vi "main_serce.vi"() -> ()   [LabVIEW 2025]
uses:
  <vilib>/Analysis/8numeric.llb/1D Numeric Integration.vi
  <vilib>/Analysis/NI_AALPro.lvlib
panel:
  out "Data unsaved!":bool
  in  "Save Data":bool
  out "CO value calculated":dbl
  out "Blood temp":dbl
  in  "CO":bool
  out "Waveform Chart":waveform(dbl)(graph)
  out "Bolus Temp":dbl
  in  "Get bolus temp":bool
  in  "Start Measurement":bool
  in  "stop (F)":bool
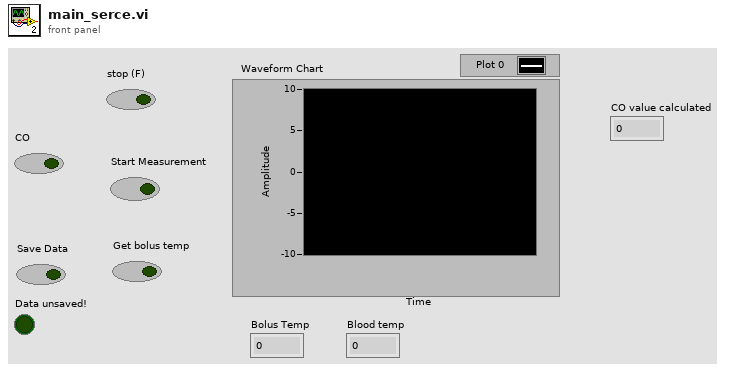
[diagram p1: front panel]
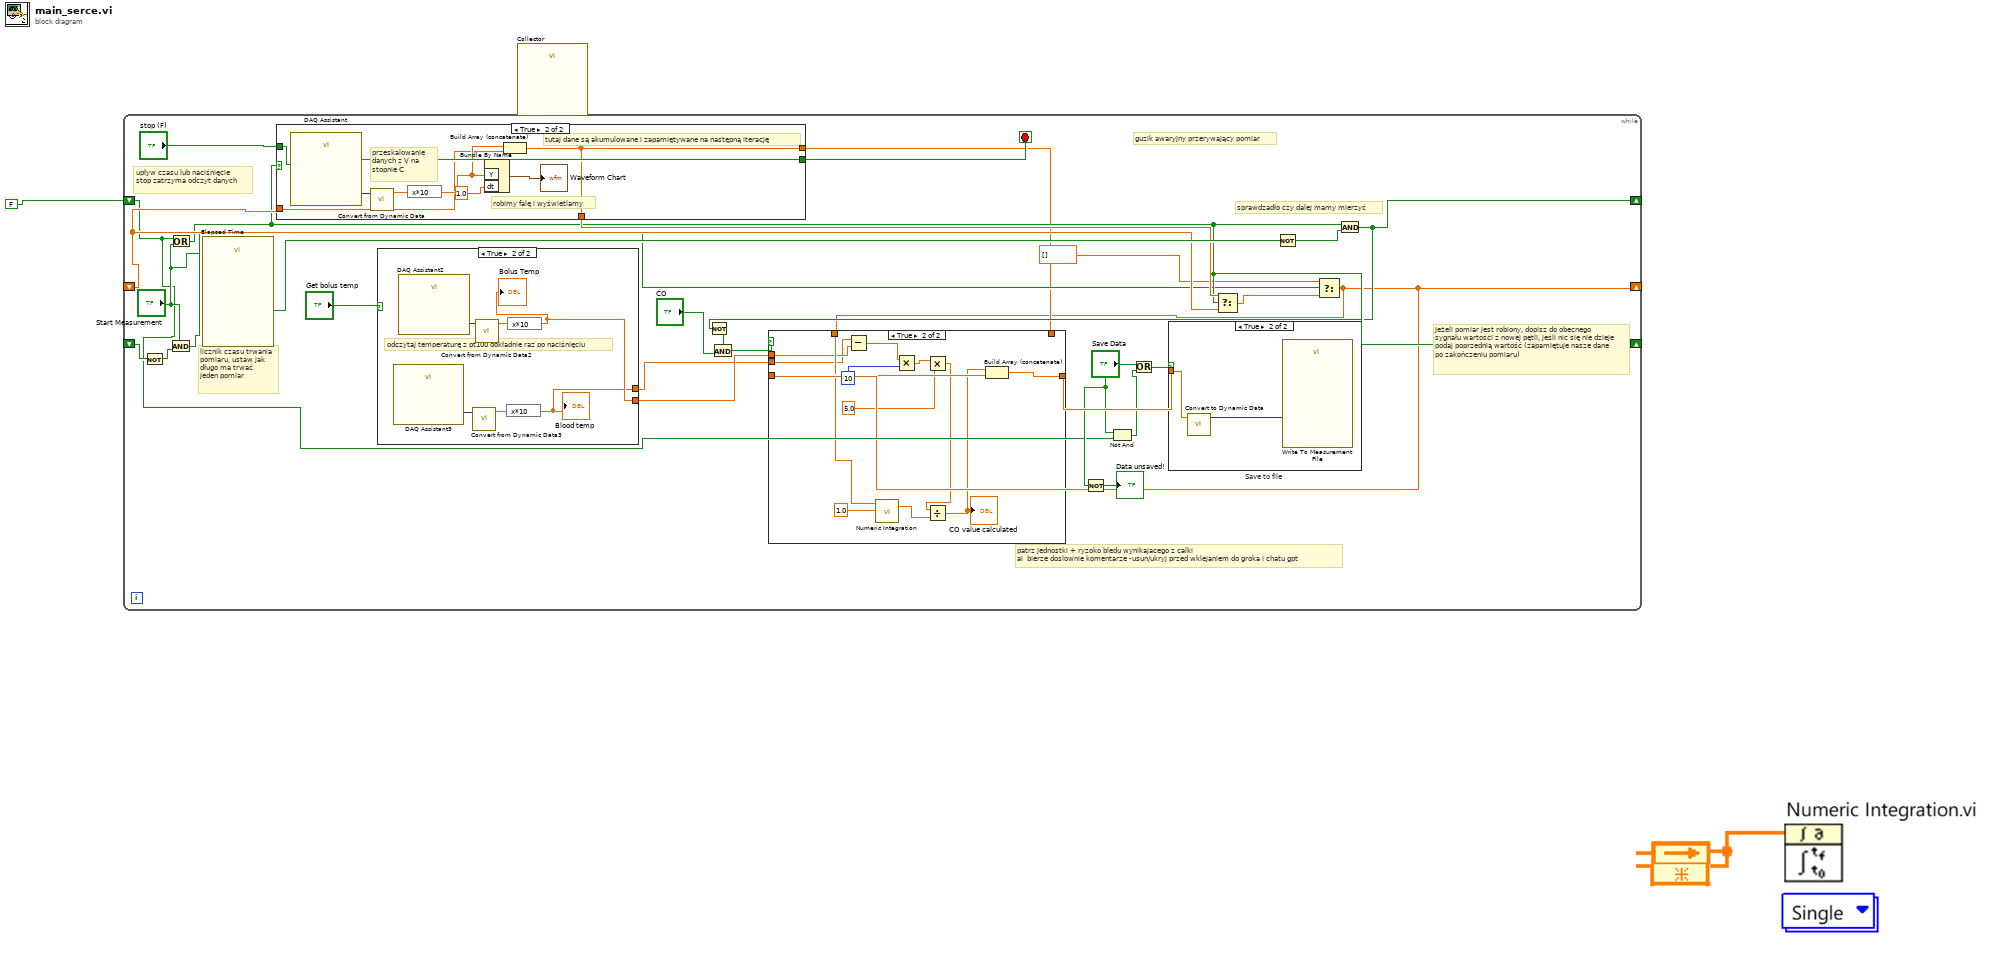
[diagram p0: block diagram]
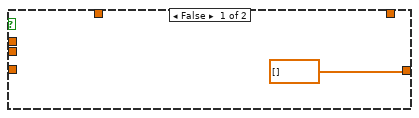
[diagram p3: hidden frame]
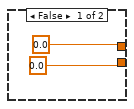
[diagram p4: hidden frame]
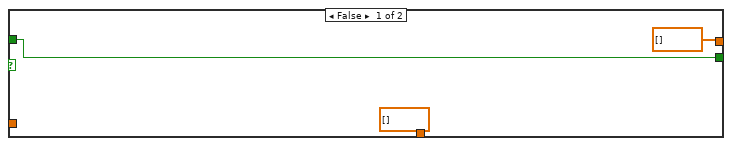
[diagram p5: hidden frame]
diagram:
  n1 = while {
    shift-right: [w16] -> _
    shift-left: FALSE -> [w5]
    shift-right: [w4] -> _
    shift-left: _ -> [w24]
    shift-right: [w23] -> _
    shift-left: _ -> [w20]
    stop <- w29 stop-if-true
    # "patrz jednostki + ryzoko bledu wynikajacego z calki \nai  bierze doslownie komentarze -usun/ukryj przed wklejaniem do groka i chatu gpt"
    # "sprawdzadło czy dalej mamy mierzyć"
    # "guzik awaryjny przerywający pomiar"
    # "Jeżeli pomiar jest robiony, dopisz do obecnego sygnału wartości z nowej pętli, jeśli nic się nie dzieje podaj poprzednią wartość (zapamiętuje nasze dane po zakończeniu pomiaru)"
    # "upływ czasu lub naciśnięcie stop zatrzyma odczyt danych"
    # "licznik czasu trwania pomiaru, ustaw jak długo ma trwać jeden pomiar"
    n2 = Not(x=w20) -> (.not. x?=w21:bool)
    n3 = And(x="Start Measurement", y=w21) -> (x .and. y?=w19:bool)
    n4 = Or(x=w5, y="Start Measurement") -> (x .or. y?=w23:bool)
    n5 = call "Elapsed Time"("Reset"="Start Measurement") -> ("Time has Elapsed"=w28:bool)  [unwired: 11 in, 7 out]
    n6 = case shown="True" w23 {
      tunnel: [w54 w65] -> w29
      tunnel: "stop (F)" -> [w54 w64]
      tunnel: w24 -> [_ w59]
      tunnel: [dbl[] [] w58] -> w25
      tunnel: [dbl[] [] w58] -> w13
      frame False {
      }
      frame True {
        # "tutaj dane są akumulowane i zapamiętywane na następną iterację"
        # "robimy falę i wyświetlamy"
        # "przeskalowanie danych z V na stopnie C"
        n7 = call "DAQ Assistant"("stop (F)"=w64) -> ("data"=w63:dynamicdata, "stopped"=w65:bool)  [unwired: 15 in, 2 out]
        n8 = call "Convert from Dynamic Data"("Dynamic Data Type"=w63) -> ("Array"=w62:dbl[])  [unwired: 3 in]
        n9 = expression code="x*10"(w62) -> (w60:dbl[])
        n10 = Bundle By Name("Y"=w60, "dt"=1.0) -> (→"Waveform Chart":waveform(dbl))  [unwired: 1 in]
        n11 = Build Array (concatenate)(w60, w59) -> (w58:dbl[])
      }
    }
    n12 = case shown="True" "Get bolus temp" {
      tunnel: [0.0 ("Scalar") w48] -> w2
      tunnel: [0.0 ("Scalar") w49] -> w3
      frame False {
      }
      frame True {
        # "odczytaj temperaturę z pt100 dokładnie raz po naciśnięciu"
        n13 = call "DAQ Assistant3"() -> ("data"=w51:dynamicdata)  [unwired: 17 in, 2 out]
        n14 = call "DAQ Assistant2"() -> ("data"=w53:dynamicdata)  [unwired: 17 in, 2 out]
        n15 = call "Convert from Dynamic Data3"("Dynamic Data Type"=w51) -> ("Scalar"=w50:dbl)  [unwired: 3 in]
        n16 = call "Convert from Dynamic Data2"("Dynamic Data Type"=w53) -> ("Scalar"=w52:dbl)  [unwired: 3 in]
        n17 = expression code="x*10"(w50) -> (w48:dbl)
        "Blood temp" <- w48
        n18 = expression code="x*10"(w52) -> (w49:dbl)
        "Bolus Temp" <- w49
      }
    }
    n19 = Not(x="Save Data") -> (.not. x?=→"Data unsaved!":bool)
    n20 = Not And(1:w5, 2:"Save Data") -> (0:w9:bool)
    n21 = Or(x="Save Data", y=w9) -> (x .or. y?=w10:bool)
    n22 = Select(t=w25, s=w23, f=w24) -> (s? t:f=w22:dbl[])
    n23 = Not(x=w28) -> (.not. x?=w27:bool)
    n24 = Select(t=dbl[] [], s=w19, f=w22) -> (s? t:f=w4:dbl[])
    n25 = And(x=w23, y=w27) -> (x .and. y?=w16:bool)
    n26 = Not(x=w16) -> (.not. x?=w14:bool)
    n27 = And(x=w14, y="CO") -> (x .and. y?=w17:bool)
    n28 = case shown="True" w17 {
      tunnel: w13 -> [_ _]
      tunnel: [dbl[] [] w45] -> w12
      tunnel: w4 -> [_ w44]
      tunnel: w4 -> [_ w36]
      tunnel: w3 -> [_ w35]
      tunnel: w2 -> [_ w34]
      frame False {
      }
      frame True {
        n29 = Subtract(x=w34, y=w35) -> (x-y=w41:dbl)
        n30 = call-poly <vilib>:"Numeric Integration.vi"("dt"=1.0, "Input Array"=w36) -> ("result"=w40:dbl)  [unwired: 1 in, 1 out]
        n31 = Multiply(x=w41, y=10) -> (x*y=w42:dbl)
        n32 = Multiply(x=w42, y=5.0 ("dt")) -> (x*y=w43:dbl)
        n33 = Divide(x=w43, y=w40) -> (x/y=w33:dbl)
        "CO value calculated" <- w33
        n34 = Build Array (concatenate)(w33, w44) -> (w45:dbl[])
      }
    }
    n35 = case "Save to file" shown="True" w10 {
      tunnel: w12 -> [_ w31]
      frame False {
      }
      frame True {
        n36 = call "Convert to Dynamic Data"("Array"=w31) -> ("Dynamic Data Type"=w30:dynamicdata)  [unwired: 3 in]
        n37 = call "Write To Measurement File"("Signals"=w30) -> ()  [unwired: 16 in, 3 out]
      }
    }
  }
  n38 = call "Collector"() -> ()  [unwired: 10 in, 2 out]
